vi "displayConfigurableElements.vi"(11 "ConfigurationThisComponent in":refnum<class "ConfigurationThisComponent.lvclass">) -> (3 "ConfigurationThisComponent out":refnum<class "ConfigurationThisComponent.lvclass">)   [LabVIEW 2015, in "ConfigurationThisComponent.lvclass"]
uses:
  ConfigurationThisComponent.lvclass
  <userlib>/Common/ILC/Configuration/Serial.ctl
  <userlib>/Common/SerialProtocols/Configuration/SerialConfig.ctl
  <userlib>/Common/SerialProtocols/Configuration/SerialProtocol.ctl
  <userlib>/Common/SerialProtocols/Configuration/ProtocolParameters.ctl
  <userlib>/Common/SerialProtocols/Configuration/SerialMessageParameters.ctl
  <userlib>/Common/Devices/DistanceGauge/Config/DistanceGauge.ctl
  <userlib>/Common/Devices/DistanceGauge/Config/ChannelsToRead.ctl
  Configuration/SystemController.ctl
  <userlib>/Common/ILC/Configuration/ADC Conversion Settings.ctl
  Configuration/StiffnessCalculator.ctl
  Model/ApplicationElements/StiffnessCalculator/Preconditioning.ctl
  <userlib>/Common/ILC/Configuration/DAC Settings.ctl
  <userlib>/Common/ILC/Configuration/ADC Collection Settings.ctl
  <userlib>/Common/ILC/Configuration/Input Channels.ctl
  <userlib>/Common/ILC/Configuration/Scan Rates.ctl
  <userlib>/Common/SerialProtocols/SerialProtocols.lvlib
  <userlib>/Common/ILC/Configuration/ILCConfiguration.lvlib
  <userlib>/Common/Devices/DistanceGauge/DistanceGauge.lvlib
panel:
  in  "ctrlRefArrayUsrEvnt":refnum<user-event>
  in  "ConfigTab":T1(tab)
  in  "ILCSerial":T2={"Serial"={"Serial Protocol"=enum."RS485", "Protocol Parameters"={"VISA resource name"="", "Baud Rate"=9600, "Data Bits"=8, "Parity"=enum."None", "Flow Control"=0, "Stop Bits"=10, "Timeout (ms)"=10000}, "Serial Message Parameters"={"Byte Count"=200, "Enable Termination Character"=FALSE, "Termination Char"=200}}} {"Serial"."Serial Message Parameters"."Termination Char" format="%x"; "Serial"."Protocol Parameters"."Stop Bits" items=["1.0"=10, "1.5"=15, "2.0"=20]; "Serial"."Protocol Parameters"."Flow Control" items=["None", "XON/XOFF", "RTS/CTS", "XON/XOFF & RTS/CTS", "DTR/DSR", "XON/XOFF & DTR/DSR"]; "Serial"."Protocol Parameters"."Data Bits" min=5 max=8 step=1}
  in  "ADC Collection Settings":T7 {"PGA Gain Coefficient" max=7}
  in  "ADC Conversion Settings":T10={"Reference Voltage Vref"=0.0, "Nominal Input Range in Counts"=128, "Preamplifier Gain (K1 * K2)"=0.0, "Conversion Settling Cycles"=0, "Excitation Voltage Vexc"=0.0} {"Excitation Voltage Vexc" min=-10.0 max=10.0 format="%.3f"; "Conversion Settling Cycles" min=1; "Preamplifier Gain (K1 * K2)" min=1.0 format="%.2f"; "Nominal Input Range in Counts" min=128; "Reference Voltage Vref" min=-10.0 max=10.0 format="%.3f"}
  in  "DAC Settings":T11={"Voltage Reference"=4.096, "Min Counts"=0, "Max Counts"=65535} {"Voltage Reference" format="%.3f"}
  in  "DistanceGauge":T12={"Serial"={"Serial Protocol"=enum."RS485", "Protocol Parameters"={"VISA resource name"="", "Baud Rate"=9600, "Data Bits"=8, "Parity"=enum."None", "Flow Control"=0, "Stop Bits"=10, "Timeout (ms)"=10000}, "Serial Message Parameters"={"Byte Count"=200, "Enable Termination Character"=FALSE, "Termination Char"=200}}, "Channels To Read"=[]} {"Serial"."Serial Message Parameters"."Termination Char" format="%x"; "Serial"."Protocol Parameters"."Stop Bits" items=["1.0"=10, "1.5"=15, "2.0"=20]; "Serial"."Protocol Parameters"."Flow Control" items=["None", "XON/XOFF", "RTS/CTS", "XON/XOFF & RTS/CTS", "DTR/DSR", "XON/XOFF & DTR/DSR"]; "Serial"."Protocol Parameters"."Data Bits" min=5 max=8 step=1}
  in  "Force Sensor Calculator":T14={"Capacity"=1.0, "Sensitivity"=0.001} {"Sensitivity" min=0.001 max=5000.0 format="%.5f"; "Capacity" min=1.0 max=5000000.0 format="%.4f"}
  in  "Preconditioning":T15 {"Number of Preconditioning Cycles" min=1 max=50}
  in  "System Controller":T16={"PreconditioningRamp Rate (%/s)"=2.0, "Stiffness Test Ramp Rate (%/s)"=2.0, "Preconditioning Ramp Target"={"Displacement"=1e-09}, "Preconditioning Ramp Safety Limit"={"Force"=0.44482220000000006}, "Stiffness Test Ramp Targets"={"Displacement"=1e-09, "Target Force"=5000.0}, "Settling"={"Displacement Max StDev"=1e-10, "Evaluation Time"=2.0}} {"Preconditioning Ramp Safety Limit"."Force" min=0.44482220000000006 max=2224.1110000000003 format="%.1f"; "Stiffness Test Ramp Rate (%/s)" min=0.001 max=50.0 format="%.1f"; "Settling"."Evaluation Time" min=0.001 max=4.0 format="%.1f"; "Settling"."Displacement Max StDev" min=2.54e-08 max=5.08 format="%.5f"; "Stiffness Test Ramp Targets"."Target Force" min=44.482220000000005 max=1779.289 format="%.1f"; "Stiffness Test Ramp Targets"."Displacement" min=0.00254 max=0.017779999999999997 format="%.1f"; "Preconditioning Ramp Target"."Displacement" min=0.00254 max=0.015239999999999998 format="%.1f"; "PreconditioningRamp Rate (%/s)" min=0.001 max=50.0 format="%.1f"}
  in  "Stiffness Calculator":T17 {"Forces in Stiffness Summary" min=44.482220000000005 max=1779.2888}
  # "Gain is 2^gain_coefficient"
  # "defined at capacity"
  # "over"
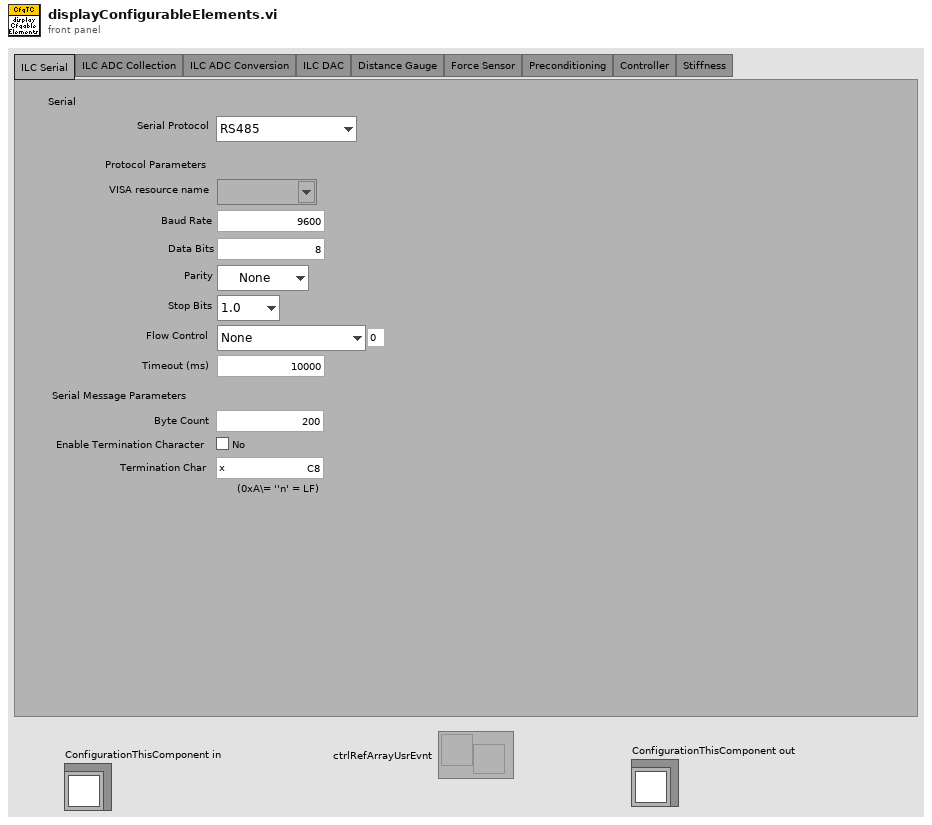
[diagram p1: front panel]
types:
  T1 = enum32{"ILC Serial", "ILC ADC Collection", "ILC ADC Conversion", "ILC DAC", "Distance Gauge", "Force Sensor", "Preconditioning", "Controller", "Stiffness"}
  T2 = typedef "ILCCommon.lvlib/ILCConfiguration.lvlib/Serial.ctl" = cluster{"Serial":T3}
  T3 = typedef "SerialProtocols.lvlib/SerialConfig.ctl" = cluster{"Serial Protocol":T4, "Protocol Parameters":T5, "Serial Message Parameters":T6}
  T4 = typedef "SerialProtocols.lvlib/SerialProtocol.ctl" = enum16{"RS232", "RS485", "SerialSimulator"}
  T5 = typedef "SerialProtocols.lvlib/ProtocolParameters.ctl" = cluster{"VISA resource name":refnum<visa-resource-name>, "Baud Rate":u32, "Data Bits":u16, "Parity":enum16{"None", "Odd", "Even", "Mark", "Space"}, "Flow Control":u16, "Stop Bits":u16, "Timeout (ms)":u32}
  T6 = typedef "SerialProtocols.lvlib/SerialMessageParameters.ctl" = cluster{"Byte Count":u32, "Enable Termination Character":bool, "Termination Char":u8}
  T7 = typedef "ILCCommon.lvlib/ILCConfiguration.lvlib/ADC Collection Settings.ctl" = cluster{"Input Channels":T8, "Scan Rate (Hz) ":T9, "PGA Gain Coefficient":u8}
  T8 = typedef "ILCCommon.lvlib/ILCConfiguration.lvlib/Input Channels.ctl" = enum16{"Channel 0", "3 Channels", "5 Channels"}
  T9 = typedef "ILCCommon.lvlib/ILCConfiguration.lvlib/Scan Rates.ctl" = enum16{"50", "60", "100", "120", "200", "240", "300", "400", "480", "600", "1200", "2400", "4800"}
  T10 = typedef "ILCCommon.lvlib/ILCConfiguration.lvlib/ADC Conversion Settings.ctl" = cluster{"Reference Voltage Vref":dbl[unit], "Nominal Input Range in Counts":u32, "Preamplifier Gain (K1 * K2)":dbl, "Conversion Settling Cycles":u16, "Excitation Voltage Vexc":dbl[unit]}
  T11 = typedef "ILCCommon.lvlib/ILCConfiguration.lvlib/DAC Settings.ctl" = cluster{"Voltage Reference":dbl[unit], "Min Counts":i32, "Max Counts":i32}
  T12 = typedef "DistanceGauge.lvlib/DistanceGauge.ctl" = cluster{"Serial":T3, "Channels To Read":T13}
  T13 = typedef "DistanceGauge.lvlib/ChannelsToRead.ctl" = i32[]
  T14 = cluster{"Capacity":dbl[unit], "Sensitivity":dbl[unit]}
  T15 = typedef "Preconditioning.ctl" = cluster{"Number of Preconditioning Cycles":u32}
  T16 = typedef "SystemController.ctl" = cluster{"PreconditioningRamp Rate (%/s)":dbl[unit], "Stiffness Test Ramp Rate (%/s)":dbl[unit], "Preconditioning Ramp Target":cluster{"Displacement":dbl[unit]}, "Preconditioning Ramp Safety Limit":cluster{"Force":dbl[unit]}, "Stiffness Test Ramp Targets":cluster{"Displacement":dbl[unit], "Target Force":dbl[unit]}, "Settling":cluster{"Displacement Max StDev":dbl[unit], "Evaluation Time":dbl[unit]}}
  T17 = typedef "StiffnessCalculator.ctl" = cluster{"Forces in Stiffness Summary":dbl[unit][]}
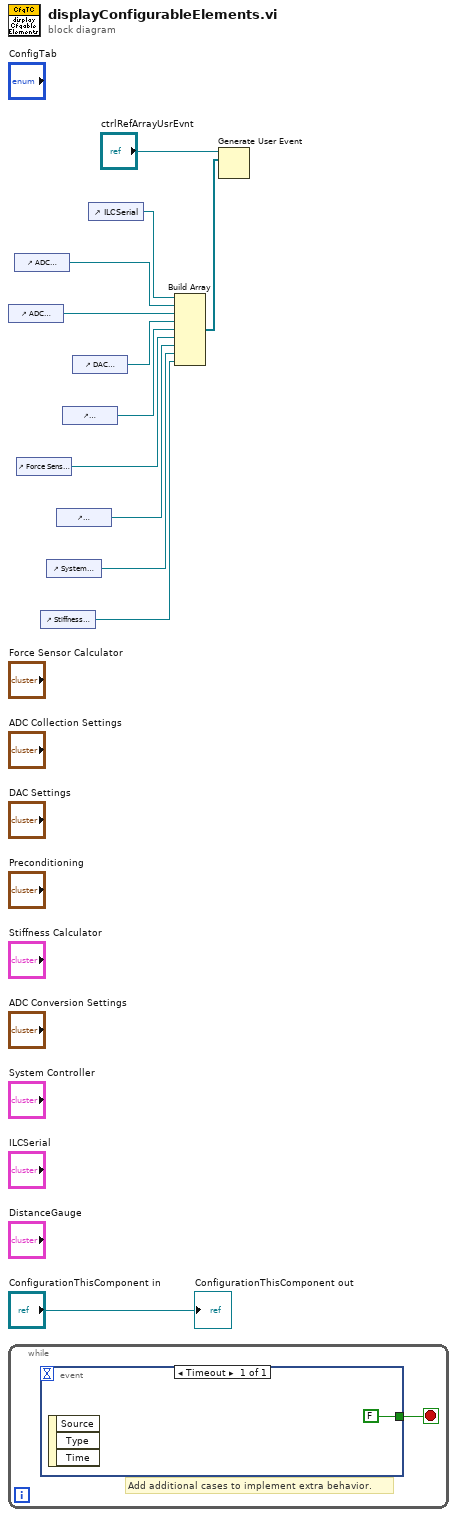
[diagram p0: block diagram]
diagram:
  n1 = control-ref of="ADC Conversion Settings"() -> (w3:refnum<vi>)
  n2 = while {
    stop <- w13 stop-if-true
    # "Add additional cases to implement extra behavior."
    n3 = event shown="[0] Timeout" {
      selector: _ -> [_]
      dyn-events: _ -> [_]
      timeout: _ -> [_]
      tunnel: [FALSE] -> w13
      event Timeout {
        n4 = event-data() -> ()  [unwired: 1 in, 3 out]
      }
    }
  }
  n5 = control-ref of="ADC Collection Settings"() -> (w2:refnum<vi>)
  n6 = control-ref of="Force Sensor Calculator"() -> (w1:refnum<vi>)
  n7 = control-ref of="Stiffness Calculator"() -> (w5:refnum<vi>)
  n8 = control-ref of="System Controller"() -> (w7:refnum<vi>)
  n9 = control-ref of="Preconditioning"() -> (w6:refnum<vi>)
  n10 = control-ref of="DistanceGauge"() -> (w8:refnum<vi>)
  n11 = control-ref of="DAC Settings"() -> (w4:refnum<vi>)
  n12 = control-ref of="ILCSerial"() -> (w9:refnum<vi>)
  n13 = Build Array(w9, w2, w3, w4, w8, w1, w6, w7, w5) -> (w12:refnum<vi>[])
  n14 = Generate User Event(user event="ctrlRefArrayUsrEvnt", event data cluster=w12) -> ()  [unwired: 2 in, 2 out]
  "ConfigurationThisComponent out" <- "ConfigurationThisComponent in"
